vi "Abstract Interface Wizard.vi"   [LabVIEW 2015]
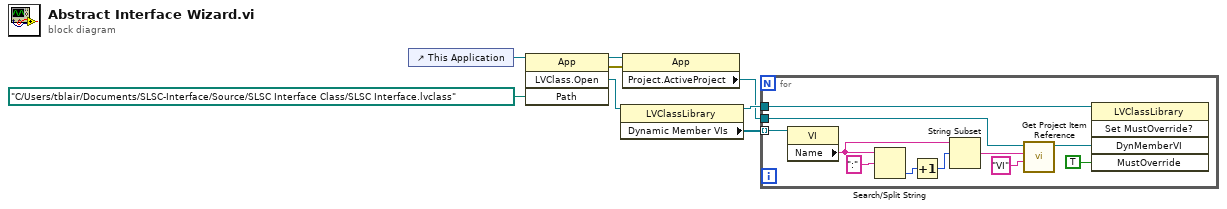
[diagram p0: block diagram]
diagram:
  n1 = control-ref of="This Application"() -> (w8:refnum<vi>)
  n2 = invoke class="App" method="LVClass.Open"(reference=w8, "Path"=path "C:/Users/tblair/Documents/SLSC-Interface/Source/SLSC Interface Class/SLSC Interface.lvclass" ("class path")) -> (reference out=w4:refnum<vi>, error out=w3:errorcluster, "LVClass.Open"=w7:refnum<vi>)  [unwired: 2 in, 1 out]
  n3 = property class="LVClassLibrary"(reference=w7) -> (reference out=w5:refnum<vi>, "Dynamic Member VIs"=w6:refnum<vi>[])  [unwired: 1 in, 1 out]
  n4 = property class="App"(reference=w4, error in=w3) -> ("Project.ActiveProject"=w2:refnum<vi>)  [unwired: 2 out]
  n5 = for {
    tunnel: w6 -> [w14] mode=indexing
    tunnel: w5 -> [w15]
    tunnel: w2 -> [w11]
    n6 = property class="VI"(reference=w14) -> ("Name"=w19:string)  [unwired: 1 in, 2 out]
    n7 = Search/Split String(string=w19, search string/char (-)=":") -> (offset of match=w17:i32)  [unwired: 1 in, 2 out]
    n8 = Increment(x=w17) -> (x+1=w16:i32)
    n9 = String Subset(string=w19, offset (0)=w16) -> (substring=w12:string)  [unwired: 1 in]
    n10 = call "Get Project Item Reference.vi"("Type"="VI", "Name"=w12, "Project Refnum"=w11) -> ("ProjectItem Refnum"=w10:refnum<vi>)  [unwired: 6 in, 2 out]
    n11 = invoke class="LVClassLibrary" method="Set MustOverride?"(reference=w15, "DynMemberVI"=w10, "MustOverride"=TRUE ("Must Override?")) -> ()  [unwired: 2 in, 5 out]
  }
